vi "SS_Wait4HistorianOK.vi"(6 "Main Cluster IN":T1, 8 "Error In":errorcluster, 11 "Info In":string="\nWaiting for TimerScope Trigger\n- IN: SS TimerScope Trigger\n- OUT: SET SS ThermoRec Received Trigger\nPulse Number is 231123\nPulse Type is 4\n\nDuration (s) is  2.000000\nDelay (s)  is  1.000000\nScan Period (ms) is  15\nNumber of Samples is  134\n\nDelay Started\nDelay Complete\nExternal Measurement of Delay (s): 1.000000\nACQUIRING DATA") -> (0 "Error Out":errorcluster, 3 "Info Out":string="\nWaiting for TimerScope Trigger\n- IN: SS TimerScope Trigger\n- OUT: SET SS ThermoRec Received Trigger\nPulse Number is 231123\nPulse Type is 4\n\nDuration (s) is  2.000000\nDelay (s)  is  1.000000\nScan Period (ms) is  15\nNumber of Samples is  134\n\nDelay Started\nDelay Complete\nExternal Measurement of Delay (s): 1.000000\nACQUIRING DATA", 4 "Main Cluster OUT":T1)   [LabVIEW 2016]
uses:
  Control/Control_Main.ctl
  Control/Control_ModuleArray.ctl
  <vilib>/Platform/TimedLoop/XDataNode/timing_clust.ctl
  <vilib>/Platform/TimedLoop/XDataNode/nitl_modes.ctl
  <vilib>/Platform/TimedLoop/XDataNode/wakeup.ctl
  <vilib>/Platform/TimedLoop/XDataNode/XDataNode.xnode
  <vilib>/Platform/TimedLoop/XDataNode/XDNodeRunTimeDep.lvlib
panel:
  in  "Tab Control":enum32{"IN", "OUT", "SubVI Info"}(tab)
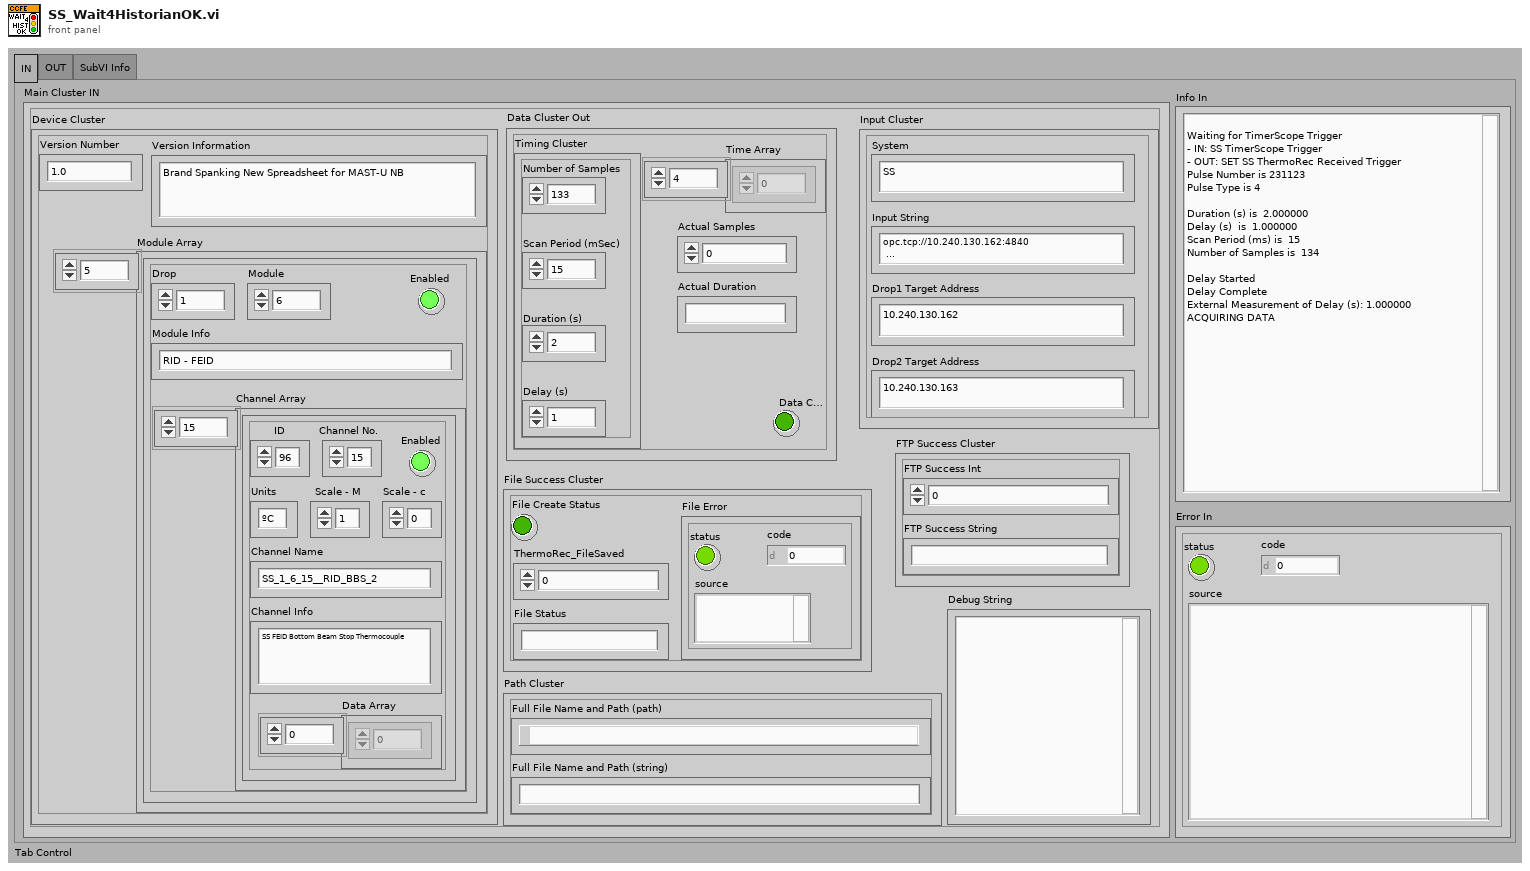
[diagram p1: front panel]
types:
  T1 = typedef "Control_Main.ctl" = cluster{"Device Cluster":cluster{"Module Array":T2, "Version Number":string, "Version Information":string}, "Input Cluster":cluster{"Input String":string, "Drop1 Target Address":string, "Drop2 Target Address":string, "System":string}, "Data Cluster Out":cluster{"Timing Cluster":cluster{"Number of Samples":i32, "Scan Period (mSec)":u32, "Duration (s)":dbl, "Delay (s)":dbl}, "Time Array":dbl[], "Actual Samples":i32, "Actual Duration":string, "Data Collection Error":bool}, "Path Cluster":cluster{"Full File Name and Path (path)":path, "Full File Name and Path (string)":string}, "File Success Cluster":cluster{"ThermoRec_FileSaved":i32, "File Create Status":bool, "File Error":errorcluster, "File Status":string}, "FTP Success Cluster":cluster{"FTP Success Int":i32, "FTP Success String":string}, "Debug String":string}
  T2 = typedef "Control_ModuleArray.ctl" = cluster{"Drop":i32, "Module":i32, "Module Info":string, "Enabled":bool, "Channel Array":cluster{"ID":i32, "Channel No.":i32, "Enabled":bool, "Channel Name":string, "Channel Info":string, "Units":string, "Scale - M":dbl, "Scale - c":dbl, "Data Array":dbl[]}[]}[]
  T3 = typedef "XDNodeRunTimeDep.lvlib/timing_clust.ctl" = cluster{"Expected End [f-1]":u64, "Actual End [f-1]":u64, "Finished Late? [f-1]":bool, "Expected End [i-1]":u64, "Actual End [i-1]":u64, "Finished Late? [i-1]":bool, "Expected Start [i]":u64, "Actual Start [i]":u64, "Expected Start [f]":u64, "Actual Start [f]":u64, "Source Name":string, "Structure Name":string, "Period":i64, "Deadline":i64, "Offset":i64, "Start":i64, "Priority":i32, "Timeout":i32, "Mode":T4, "Wakeup Reason":T5, "Error":errorcluster, "Source Type":string, "Secondary Source Type":string, "Global End Time":u64, "Global Start Time":u64, "Frame Duration":u64, "Iteration Duration":u64, "Assigned CPU":i32, "I/O Scan Engine Mode":u32}
  T4 = typedef "XDNodeRunTimeDep.lvlib/nitl_modes.ctl" = enum32{"No Change", "Process missed periods, maintain original phase", "Discard missed periods, maintain original phase", "Process missed periods, ignore original phase", "Discard missed periods, ignore original phase"}
  T5 = typedef "XDNodeRunTimeDep.lvlib/wakeup.ctl" = enum32{"Normal", "Aborted", "Asynchronous wakeup", "Timing source error", "Timed loop error", "Timeout"}
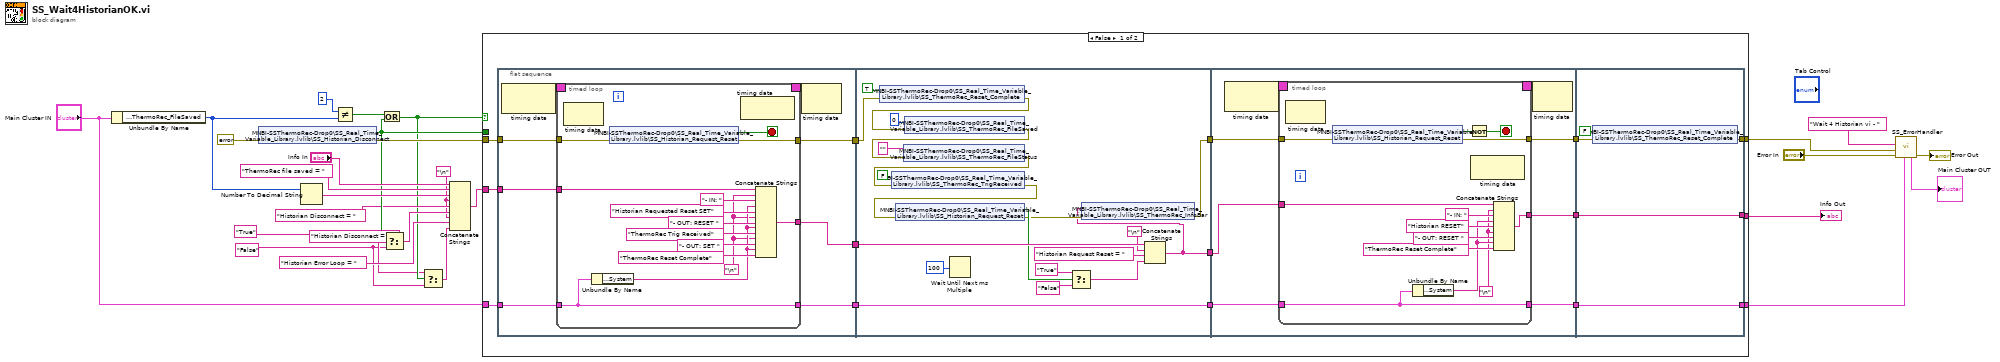
[diagram p0: block diagram]
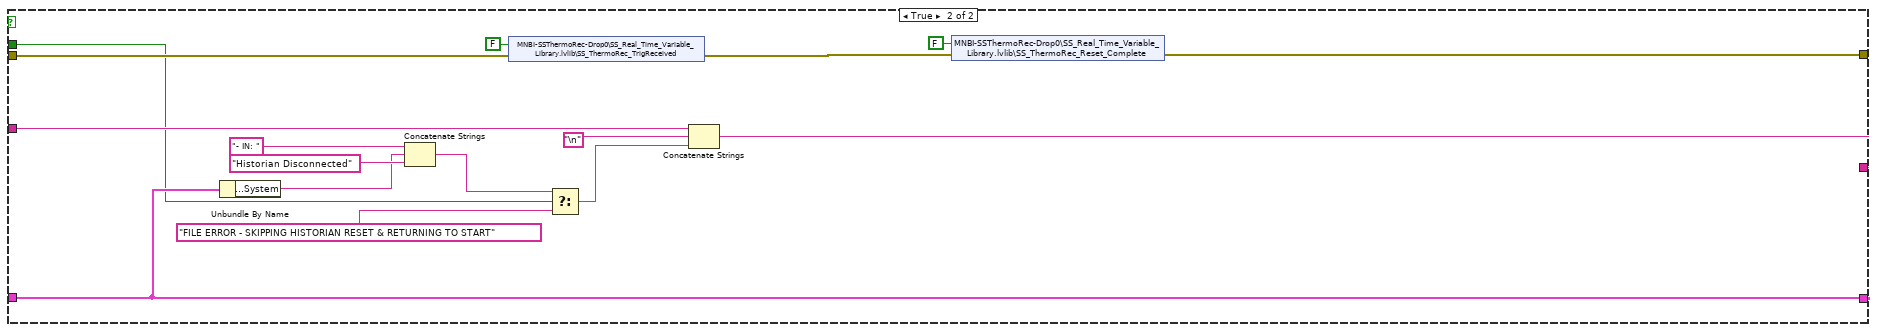
[diagram p2: hidden frame]
diagram:
  (unwired) "Historian Disconnect = "
  w5 = "False"
  w6 = "True"
  w9 = "\n"
  n1 = Unbundle By Name("Main Cluster IN") -> ("File Success Cluster.ThermoRec_FileSaved"=w2:i32)
  n2 = shared-variable "MNBI-SSThermoRec-Drop0\\SS_Real_Time_Variable_Library.lvlib\\SS_Historian_Disconnect"(error in=errorcluster {"status"=FALSE, "code"=0, "source"=""} ("error constant")) -> (w12:bool, error out=w24:errorcluster)
  n3 = Number To Decimal String(number=w2) -> (decimal integer string=w13:string)  [unwired: 1 in]
  n4 = Not Equal?(x=2, y=w2) -> (x != y?=w25:bool)
  n5 = Or(x=w25, y=w12) -> (x .or. y?=w7:bool)
  n6 = Select(t=w6, s=w12, f=w5) -> (s? t:f=w10:string)
  n7 = Select(t=w6, s=w7, f=w5) -> (s? t:f=w4:string)
  n8 = Concatenate Strings("Info In", "ThermoRec file saved = ", w13, w9, "Historian Disconnect = ", w10, w9, "Historian Error Loop = ", w4) -> (w15:string)
  n9 = case shown="False" w7 {
    tunnel: w24 -> [w41 w126]
    tunnel: w15 -> [w40 w134]
    tunnel: [w29 w129] -> w18
    tunnel: [w28 w132] -> w22
    tunnel: "Main Cluster IN" -> [w39 w125]
    tunnel: [w27 w125] -> w17
    tunnel: w12 -> [_ w121]
    frame False {
      n10 = flat-sequence {
        tunnel: w41 -> [w47]
        tunnel: w40 -> [w46]
        tunnel: w39 -> [w43]
        tunnel: [w45] -> w38
        tunnel: [w44] -> w37
        tunnel: [w42] -> w36
        tunnel: w38 -> [w80]
        tunnel: w37 -> [w81]
        tunnel: w36 -> [w88]
        tunnel: [w68] -> w35
        tunnel: [w88] -> w34
        tunnel: [w69] -> w33
        tunnel: w35 -> [w92]
        tunnel: w34 -> [w91]
        tunnel: w33 -> [w94]
        tunnel: [w90] -> w32
        tunnel: [w89] -> w31
        tunnel: [w93] -> w30
        tunnel: [w117] -> w27
        tunnel: [w118] -> w28
        tunnel: w32 -> [w118]
        tunnel: w31 -> [w117]
        tunnel: w30 -> [w115]
        tunnel: [w114] -> w29
        frame #0 {
          n11 = node-c288() -> (w49:T3)  [unwired: 1 in]
          n12 = timed-loop {
            timing: w49 -> [_]
            timing-out: [_] -> w48
            tunnel: [w60] -> w44
            tunnel: w47 -> [w61]
            tunnel: [w63] -> w45
            tunnel: w46 -> [w62]
            tunnel: w43 -> [w57]
            tunnel: [w57] -> w42
            stop <- w59 stop-if-true
            w50 = "\n"
            n13 = node-c288() -> ()  [unwired: 1 in, 1 out]
            n14 = Unbundle By Name(w57) -> ("Input Cluster.System"=w52:string)
            n15 = shared-variable "MNBI-SSThermoRec-Drop0\\SS_Real_Time_Variable_Library.lvlib\\SS_Historian_Request_Reset"(error in=w61) -> (w59:bool, error out=w60:errorcluster)
            n16 = node-c288() -> ()  [unwired: 1 in, 1 out]
            n17 = Concatenate Strings(w62, w50, "- IN: ", w52, "Historian Requested Reset SET", w50, "- OUT: RESET ", w52, "ThermoRec Trig Received", w50, "- OUT: SET ", w52, "ThermoRec Reset Complete") -> (w63:string)
          }
          n18 = node-c288(w48) -> ()  [unwired: 1 out]
        }
        frame #1 {
          n19 = shared-variable "MNBI-SSThermoRec-Drop0\\SS_Real_Time_Variable_Library.lvlib\\SS_ThermoRec_Reset_Complete"(TRUE, error in=w81) -> (error out=w83:errorcluster)
          n20 = shared-variable "MNBI-SSThermoRec-Drop0\\SS_Real_Time_Variable_Library.lvlib\\SS_ThermoRec_FileSaved"(0 ("SS_ThermoRec_FileSaved"), error in=w83) -> (error out=w84:errorcluster)
          n21 = shared-variable "MNBI-SSThermoRec-Drop0\\SS_Real_Time_Variable_Library.lvlib\\SS_ThermoRec_FileStatus"("" ("SS_ThermoRec_FileStatus"), error in=w84) -> (error out=w85:errorcluster)
          n22 = shared-variable "MNBI-SSThermoRec-Drop0\\SS_Real_Time_Variable_Library.lvlib\\SS_ThermoRec_TrigReceived"(FALSE, error in=w85) -> (error out=w73:errorcluster)
          n23 = shared-variable "MNBI-SSThermoRec-Drop0\\SS_Real_Time_Variable_Library.lvlib\\SS_Historian_Request_Reset"(error in=w73) -> (w74:bool, error out=w70:errorcluster)
          n24 = Wait Until Next ms Multiple(millisecond multiple=u32 100) -> ()  [unwired: 1 out]
          n25 = Select(t="True", s=w74, f="False") -> (s? t:f=w75:string)
          n26 = Concatenate Strings(w80, "\n", "Historian Request Reset = ", w75) -> (w68:string)
          n27 = shared-variable "MNBI-SSThermoRec-Drop0\\SS_Real_Time_Variable_Library.lvlib\\SS_ThermoRec_InfoBar"(w68, error in=w70) -> (error out=w69:errorcluster)
        }
        frame #2 {
          n28 = node-c288() -> (w96:T3)  [unwired: 1 in]
          n29 = timed-loop {
            timing: w96 -> [_]
            timing-out: [_] -> w95
            tunnel: [w105] -> w93
            tunnel: w94 -> [w106]
            tunnel: [w107] -> w90
            tunnel: w92 -> [w108]
            tunnel: w91 -> [w103]
            tunnel: [w103] -> w89
            stop <- w109 stop-if-true
            w97 = "\n"
            n30 = node-c288() -> ()  [unwired: 1 in, 1 out]
            n31 = shared-variable "MNBI-SSThermoRec-Drop0\\SS_Real_Time_Variable_Library.lvlib\\SS_Historian_Request_Reset"(error in=w106) -> (w104:bool, error out=w105:errorcluster)
            n32 = Unbundle By Name(w103) -> ("Input Cluster.System"=w99:string)
            n33 = Not(x=w104) -> (.not. x?=w109:bool)
            n34 = node-c288() -> ()  [unwired: 1 in, 1 out]
            n35 = Concatenate Strings(w108, w97, "- IN: ", w99, "Historian RESET", w97, "- OUT: RESET ", w99, "ThermoRec Reset Complete") -> (w107:string)
          }
          n36 = node-c288(w95) -> ()  [unwired: 1 out]
        }
        frame #3 {
          n37 = shared-variable "MNBI-SSThermoRec-Drop0\\SS_Real_Time_Variable_Library.lvlib\\SS_ThermoRec_Reset_Complete"(FALSE, error in=w115) -> (error out=w114:errorcluster)
        }
      }
    }
    frame True {
      n38 = Unbundle By Name(w125) -> ("Input Cluster.System"=w122:string)
      n39 = Concatenate Strings("- IN: ", w122, "Historian Disconnected") -> (w119:string)
      n40 = shared-variable "MNBI-SSThermoRec-Drop0\\SS_Real_Time_Variable_Library.lvlib\\SS_ThermoRec_TrigReceived"(FALSE, error in=w126) -> (error out=w127:errorcluster)
      n41 = Select(t=w119, s=w121, f="FILE ERROR - SKIPPING HISTORIAN RESET & RETURNING TO START") -> (s? t:f=w131:string)
      n42 = Concatenate Strings(w134, "\n", w131) -> (w132:string)
      n43 = shared-variable "MNBI-SSThermoRec-Drop0\\SS_Real_Time_Variable_Library.lvlib\\SS_ThermoRec_Reset_Complete"(FALSE, error in=w127) -> (error out=w129:errorcluster)
    }
  }
  "Info Out" <- w22
  n44 = call "SS_ErrorHandler.vi"("Main Cluster IN"=w17, "Error In"="Error In", "SubVI Error"=w18, "SubVI Name"="Wait 4 Historian vi - ") -> ("Error Out"=→"Error Out":errorcluster, "Main Cluster OUT"=→"Main Cluster OUT":T1)  [unwired: 5 in, 1 out]
